vi "Bead Tracking Set up.vi"(8 "error in (no error)":errorcluster, 10 "SubPixel Accuracy":bool=TRUE, 11 "Template":T1) -> (0 "error out":errorcluster, 3 "Match Pattern Setup Data":string)   [LabVIEW 2011]
doc: "This VI does all the initialization work needed for bead tracking.\nIt is basically contains all the work that \"IMAQ Find Pattern 2\" (in NI_Vision_Development_Module.lvlib) does that doesn't need to be re-done between two frames."
uses:
  <vilib>/vision/Image Controls.llb/IMAQ Image.ctl
  <vilib>/vision/NI_Vision_Development_Module.lvlib
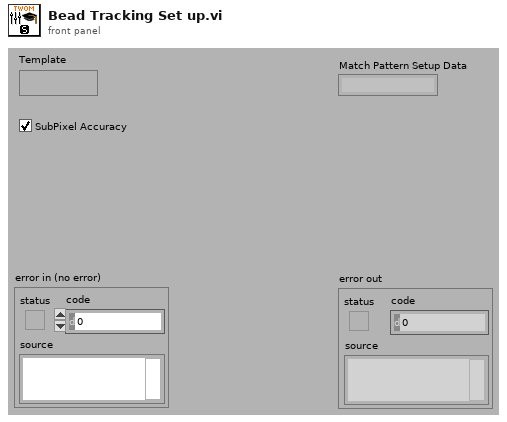
[diagram p1: front panel]
types:
  T1 = typedef "IMAQ Image.ctl" = refnum<image>
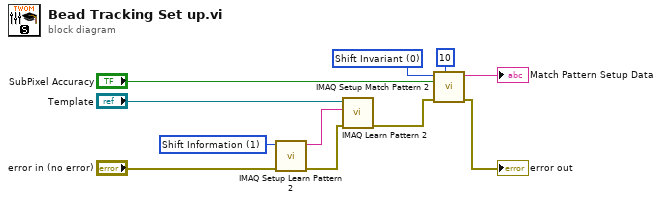
[diagram p0: block diagram]
diagram:
  w4 = u16 0 items=["Shift Invariant", "Rotation Invariant"] ("Match Mode")
  w10 = u16 1 items=["All", "Shift Information", "Rotation Information"] ("Learn Mode")
  n1 = call "IMAQ Setup Learn Pattern 2"("error in (no error)"="error in (no error)", "Learn Mode"=w10) -> ("error out"=w8:errorcluster, "Learn Pattern Setup Data"=w9:string)  [unwired: 8 out]
  n2 = call "IMAQ Learn Pattern 2"("error in (no error)"=w8, "Learn Pattern Setup Data"=w9, "Image"="Template") -> ("error out"=w6:errorcluster)  [unwired: 1 in, 7 out]
  n3 = call "IMAQ Setup Match Pattern 2"("Minimum Contrast"=10, "error in (no error)"=w6, "Subpixel Accuracy"="SubPixel Accuracy", "Match Mode"=w4) -> ("error out"=→"error out":errorcluster, "Match Pattern Setup Data"=→"Match Pattern Setup Data":string)  [unwired: 1 in, 5 out]
